vi "Load exp.vi"(7 "Window Title":string="Select Files:", 8 "error in (no error)":errorcluster, 10 "Files of Type":string[][](array[string])=[["*.dat", "DAT"], ["*.img", "Streak"], ["*.txt", "txt"], ["*.*", "All Files"]], 11 "Control-Client in":refnum<class "Control-Client.lvclass">) -> (0 "error out":errorcluster, 3 "Control-Client out":refnum<class "Control-Client.lvclass">)   [LabVIEW 2015, in "Control-Client.lvclass"]
uses:
  Control-Client.lvclass
  Control-Client.lvclass/Control-Client.ctl
  methods/Read Group #.vi
  Experiments/Experiments_group.lvclass
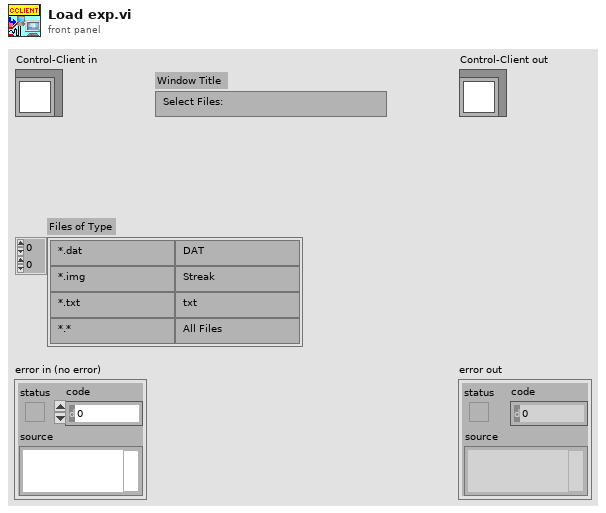
[diagram p1: front panel]
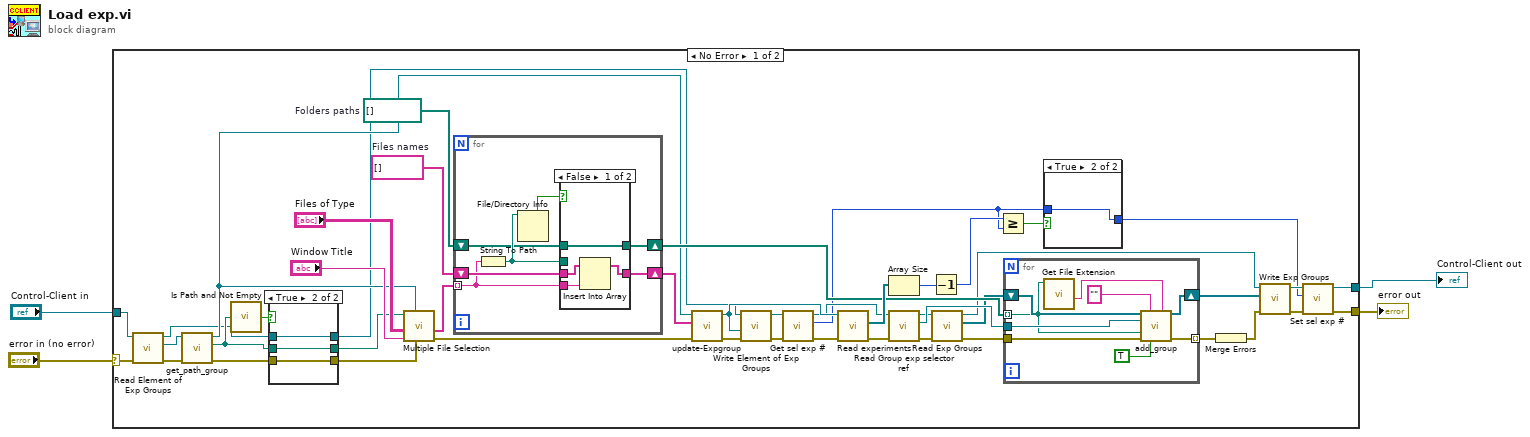
[diagram p0: block diagram]
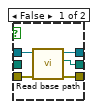
[diagram p2: hidden frame]
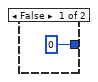
[diagram p3: hidden frame]
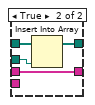
[diagram p4: hidden frame]
diagram:
  n1 = case shown="No Error" "error in (no error)" {
    selector: "error in (no error)" -> [w17 w86]
    tunnel: [w28 w86] -> w3
    tunnel: [w27 w85] -> w1
    tunnel: "Control-Client in" -> [w18 w85]
    frame No Error {
      w45 = path[] []  # Folders paths
      w44 = string[] []  # Files names
      n2 = call "Read Element of Exp Groups.vi"("error in (no error)"=w17, "Control-Client in"=w18) -> ("error out"=w12:errorcluster, "Experiments_group.lvclass"=w13:refnum<class "Experiments_group.lvclass">, "Control-Client out"=w8:refnum<class "Control-Client.lvclass">)  [unwired: 7 in]
      n3 = call "get_path_group.vi"("error in (no error)"=w12, "Experiments_group.lvclass in"=w13) -> ("error out"=w7:errorcluster, "Path"=w10:path, "Experiments_group.lvclass out"=w14:refnum<class "Experiments_group.lvclass">)  [unwired: 7 in]
      n4 = call <vilib>:"Is Path and Not Empty.vi"("path"=w10) -> ("Is Path and Not Empty?"=w11:bool)  [unwired: 4 in]
      n5 = case shown="True" w11 {
        tunnel: [w52 w58] -> w9
        tunnel: w10 -> [_ w58]
        tunnel: w8 -> [w55 w56]
        tunnel: w7 -> [w54 w57]
        tunnel: [w53 w57] -> w6
        tunnel: [w51 w56] -> w5
        frame False {
          n6 = call "Read base path.vi"("error in (no error)"=w54, "Control-Client in"=w55) -> ("error out"=w53:errorcluster, "Base path"=w52:path, "Control-Client out"=w51:refnum<class "Control-Client.lvclass">)  [unwired: 7 in]
        }
        frame True {
        }
      }
      n7 = call "Multiple File Selection.vi"("error in"=w6, "EXP group IN"=w14, "Window Title"="Window Title", "Files of Type In"="Files of Type", "Start In"=w9) -> ("error out"=w16:errorcluster, "String File Names"=w43:string[])  [unwired: 3 in, 2 out]
      n8 = for {
        tunnel: w43 -> [w72] mode=indexing
        shift-right: [w74] -> w19
        shift-left: w44 -> [w73]
        shift-right: [w70] -> w46
        shift-left: w45 -> [w71]
        n9 = String To Path(string=w72) -> (path=w76:path)
        n10 = File/Directory Info(path=w76) -> (directory=w75:bool)  [unwired: 1 in, 6 out]
        n11 = case shown="False" w75 {
          tunnel: w76 -> [_ w81]
          tunnel: [w78 w84] -> w74
          tunnel: w73 -> [w80 w84]
          tunnel: w72 -> [w79 _]
          tunnel: w71 -> [w77 w83]
          tunnel: [w77 w82] -> w70
          frame False {
            n12 = Insert Into Array(array=w80, new element=w79) -> (w78:string[])  [unwired: 1 in]
          }
          frame True {
            n13 = Insert Into Array(array=w83, new element=w81) -> (w82:path[])  [unwired: 1 in]
          }
        }
      }
      n14 = call "update-Expgroup.vi"("error in"=w16, "String File Paths"=w19, "EXP group"=w14) -> ("error out"=w37:errorcluster, "EXP group out"=w38:refnum<class "Experiments_group.lvclass">)  [unwired: 7 in]
      n15 = call "Write Element of Exp Groups.vi"("error in (no error)"=w37, "Experiments_group.lvclass"=w38, "Control-Client in"=w5) -> ("error out"=w34:errorcluster, "Control-Client out"=w35:refnum<class "Control-Client.lvclass">)  [unwired: 7 in]
      n16 = call "Get sel exp #.vi"("error in (no error)"=w34, "Control-Client in"=w35) -> ("error out"=w33:errorcluster, "Exp sel #"=w32:i32, "Control-Client out"=w36:refnum<class "Control-Client.lvclass">)  [unwired: 7 in]
      n17 = call "Read experiments.vi"("error in (no error)"=w33, "Experiments_group.lvclass in"=w38) -> ("error out"=w15:errorcluster, "Experiments"=w50:refnum<class "Experiment.lvclass">[])  [unwired: 6 in, 1 out]
      n18 = Array Size(array=w50) -> (size(s)=w47:i32)
      n19 = call "Read Group exp selector ref.vi"("error in (no error)"=w15, "Control-Client in"=w36) -> ("error out"=w23:errorcluster, "Group exp selector ref"=w39:refnum<vi>, "Control-Client out"=w26:refnum<class "Control-Client.lvclass">)  [unwired: 7 in]
      n20 = Decrement(x=w47) -> (x-1=w48:i32)
      n21 = call "Read Exp Groups.vi"("error in (no error)"=w23, "Control-Client in"=w26) -> ("error out"=w22:errorcluster, "Exp Groups"=w24:refnum<class "Experiments_group.lvclass">[], "Control-Client out"=w25:refnum<class "Control-Client.lvclass">)  [unwired: 7 in]
      n22 = Greater Or Equal?(x=w48, y=w32) -> (x >= y?=w49:bool)
      n23 = for {
        tunnel: w39 -> [w69]
        shift-right: [w65] -> w40
        shift-left: w24 -> [w66]
        tunnel: w46 -> [w63] mode=indexing
        tunnel: w22 -> [w68]
        tunnel: [w67] -> w21 mode=indexing
        n24 = call <vilib>:"Get File Extension.vi"("file"=w63) -> ("filename without extension"=w62:string)  [unwired: 6 in, 4 out]
        n25 = call "add_group.vi"("Experiments groups in"=w66, "Commentaires group"="", "Name group"=w62, "group"=w69, "Folder path"=w63, "error in (no error)"=w68, "Upload"=TRUE) -> ("Experiments groups out"=w65:refnum<class "Experiments_group.lvclass">[], "error out"=w67:errorcluster)  [unwired: 7 in]
      }
      n26 = case shown="True" w49 {
        tunnel: w32 -> [_ w60]
        tunnel: [0 w60] -> w30
        frame False {
        }
        frame True {
        }
      }
      n27 = Merge Errors(w21) -> (w20:errorcluster)
      n28 = call "Write Exp Groups.vi"("error in (no error)"=w20, "Exp Groups"=w40, "Control-Client in"=w25) -> ("error out"=w29:errorcluster, "Control-Client out"=w31:refnum<class "Control-Client.lvclass">)  [unwired: 7 in]
      n29 = call "Set sel exp #.vi"("error in (no error)"=w29, "Exp sel #"=w30, "Control-Client in"=w31) -> ("error out"=w28:errorcluster, "Control-Client out"=w27:refnum<class "Control-Client.lvclass">)  [unwired: 7 in]
    }
    frame Error {
    }
  }
  "error out" <- w3
  "Control-Client out" <- w1
